vi "Create.vi"(8 "error in (no error)":errorcluster) -> (0 "error out":errorcluster, 3 "Event Registration Refnum":refnum<event-registration>)   [LabVIEW 2017, in "WebServiceImporter.lvlib" / "Main Panel.lvlib" / "Finish.lvlib" / "Events.lvlib"]
uses:
  <vilib>/Platform/WebService/Main Panel/Pages/Finish/Events/Events.lvlib
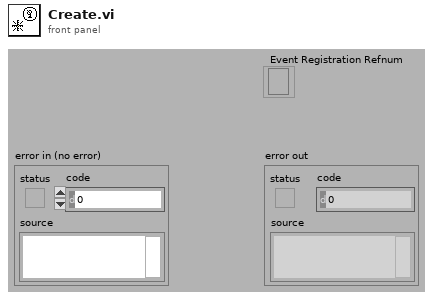
[diagram p1: front panel]
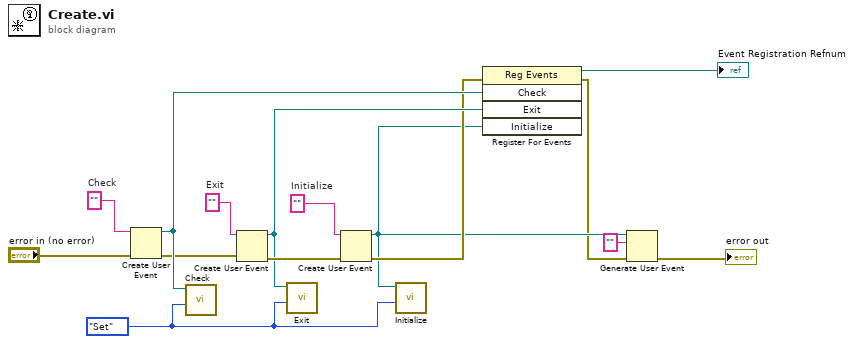
[diagram p0: block diagram]
diagram:
  w10 = ""  # Initialize
  w12 = ""  # Exit
  w7 = enum16{"Get", "Set"}."Set" ("Operation")
  w14 = ""  # Check
  n1 = Create User Event(user event datatype=w14, error in="error in (no error)") -> (user event=w13:refnum<user-event>, error out=w11:errorcluster)
  n2 = call <vilib>:"Check.vi"("Operation"=w7, "user event"=w13) -> ()  [unwired: 8 in, 2 out]
  n3 = Create User Event(user event datatype=w12, error in=w11) -> (user event=w8:refnum<user-event>, error out=w9:errorcluster)
  n4 = call <vilib>:"Exit.vi"("Operation"=w7, "user event"=w8) -> ()  [unwired: 8 in, 2 out]
  n5 = Create User Event(user event datatype=w10, error in=w9) -> (user event=w5:refnum<user-event>, error out=w6:errorcluster)
  n6 = call <vilib>:"Initialize.vi"("Operation"=w7, "user event"=w5) -> ()  [unwired: 9 in, 1 out]
  n7 = register-events(error in=w6, w13, w8, w5) -> (reference out=→"Event Registration Refnum":refnum<event-registration>, error out=w3:errorcluster)  [unwired: 1 in]
  n8 = Generate User Event(user event=w5, event data cluster="" ("event data"), error in=w3) -> (error out=→"error out":errorcluster)  [unwired: 1 in, 1 out]
